vi "x_array.vi"(9 "x0":dbl, 10 "dx":dbl, 11 "Y":dbl[](array[numeric])) -> (3 "X":dbl[](array[numeric]))   [LabVIEW 2016]
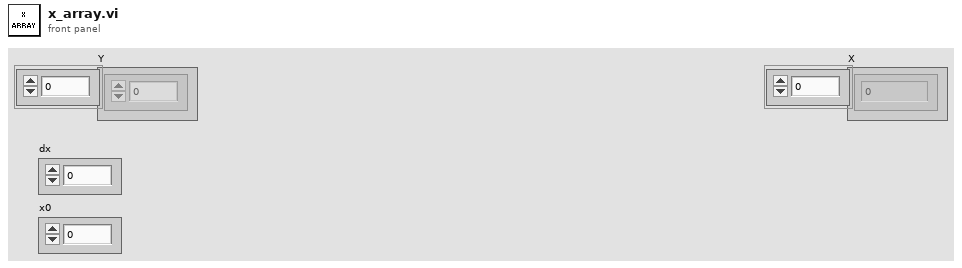
[diagram p1: front panel]
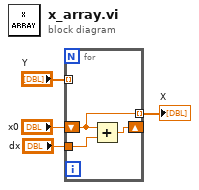
[diagram p0: block diagram]
diagram:
  n1 = for {
    shift-right: [w6] -> _
    shift-left: "x0" -> [w5]
    tunnel: "Y" -> [_] mode=indexing
    tunnel: "dx" -> [w7]
    tunnel: [w5] -> w1 mode=indexing
    n2 = Add(x=w5, y=w7) -> (x+y=w6:dbl)
  }
  "X" <- w1
